vi "user32.vi"(0 "Icon":u16(ring) items=["None", "Critical", "Question", "Exclamation", "Infomation"], 1 "Buttons":u16(ring) items=["OK", "OK+Cancel", "Abort+Retry+Ignore", "Yes+ON+Cancel", "Yes+No", "Retry+Cancel", "Cancel+Retry+Continue"], 2 "Ipcaption":string, 3 "IP Text":string) -> (4 "u Type":i32, 5 "buttin pressed":i32)   [LabVIEW 2018]
uses:
  user32.dll
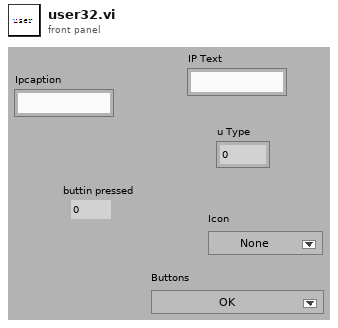
[diagram p1: front panel]
types:
  T1 = cluster{"Left Button Key Shortcut":cluster{"Control":bool, "Shift":bool, "Key":string}, "Center Button Key Shortcut":cluster{"Control":bool, "Shift":bool, "Key":string}, "Right Button Key Shortcut":cluster{"Control":bool, "Shift":bool, "Key":string}}
  T2 = enum16{"Left Button", "Center Button", "Right Button", "Window Close"}
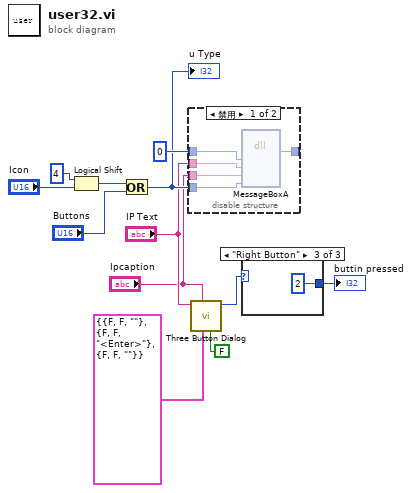
[diagram p0: block diagram]
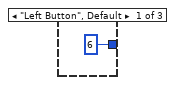
[diagram p2: hidden frame]
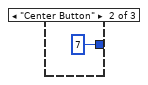
[diagram p3: hidden frame]
diagram:
  n1 = Logical Shift(y=i16 4, x="Icon") -> (x << y=w9:u16)
  n2 = Or(x=w9, y="Buttons") -> (x .or. y?=w7:u16)
  "u Type" <- w7
  n3 = disable-structure shown="禁用" {
    disable-tunnel: 0 ("Hwnd") -> [w17 _]
    disable-tunnel: w7 -> [w16 _]
    disable-tunnel: "IP Text" -> [w15 _]
    disable-tunnel: [w14 _] -> _
    disable-tunnel: "Ipcaption" -> [w13 _]
    frame Disabled {
      n4 = dll-call lib="user32.dll" fn="MessageBoxA"("Hwnd"=w17, "IP Text"=w15, "Ipcaption"=w13, "u Type"=w16) -> (w14:i32)  [unwired: 6 in, 3 out]
    }
    frame Enabled {
    }
  }
  n5 = call <vilib>:"Three Button Dialog.vi"("Allow user to close window? (TRUE)"=FALSE, "Keyboard Shortcuts (Left is <Enter>)"=T1 {"Left Button Key Shortcut"={"Control"=FALSE, "Shift"=FALSE, "Key"=""}, "Center Button Key Shortcut"={"Control"=FALSE, "Shift"=FALSE, "Key"="<Enter>"}, "Right Button Key Shortcut"={"Control"=FALSE, "Shift"=FALSE, "Key"=""}}, "Window Title (\"\")"="Ipcaption", "message"="IP Text") -> ("Which Button?"=w4:T2)  [unwired: 7 in]
  n6 = case shown="\"Right Button\"" w4 {
    tunnel: [6 7 2] -> w3
    frame "Left Button", Default {
    }
    frame "Center Button" {
    }
    frame "Right Button" {
    }
  }
  "buttin pressed" <- w3
